vi "Temperature Monitor FPGA.vi"() -> ()   [LabVIEW 2010]
uses:
  <vilib>/eio/EIONode/EIONode.xnode
panel:
  out "code":i32
  out "status":bool
  out "Autozero":fxp<+/-,24,-2> format="%.26g"
  out "CJC":fxp<+/-,24,-2> format="%.26g"
  out "Temperature":fxp<+/-,24,-2> format="%.26g"
  in  "Sample Period (ms)":u32=500
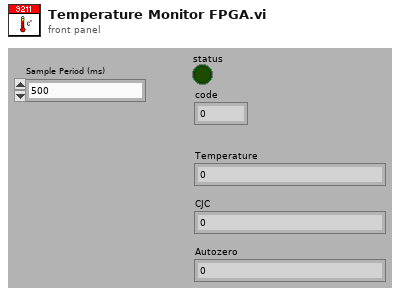
[diagram p1: front panel]
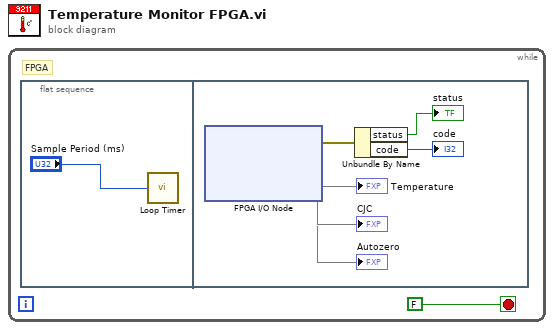
[diagram p0: block diagram]
diagram:
  n1 = while {
    stop <- FALSE stop-if-true
    # "FPGA"
    n2 = flat-sequence {
      frame #0 {
        n3 = call "Loop Timer"("Count(mSec)"="Sample Period (ms)") -> ()  [unwired: 1 out]
      }
      frame #1 {
        n4 = xnode "FPGA I/O Node"() -> ("error out"=w5:errorcluster, "Mod1/TC0"=→"Temperature", "Mod1/CJC"=→"CJC", "Mod1/Autozero"=→"Autozero")  [unwired: 4 in, 3 out]
        n5 = Unbundle By Name(w5) -> ("status"=→"status":bool, "code"=→"code":i32)
      }
    }
  }
